vi "LSMcontroller_v58.vi"() -> ()   [LabVIEW 2015] (continued)
                    n3053 = local write "status"(w6244) -> ()
                  }
                  frame #2 {
                    n3054 = call "2pparameters.vi"("command"="get") -> ("params out"=w6274:T12)  [unwired: 1 in]
                    n3055 = Unbundle By Name(w6274) -> ("Xpixels Img"=w6273:i32, "Vx-min Img"=w6272:dbl, "VX-max Img"=w6271:dbl, "Ypixels Img"=w6270:i32, "Vy-min Img"=w6269:dbl, "Vy-max Img"=w6268:dbl, "Colormap"=w6267:u16, "square pixels"=w6266:bool, "square matrix"=w6265:bool, "Angle Img"=w6264:dbl, "Drawing Mode"=w6263:u16)
                    n3056 = local write "xpixels ref"(w6273) -> ()
                    n3057 = local write "Vx-min ref"(w6272) -> ()
                    n3058 = local write "Vx-max ref"(w6271) -> ()
                    n3059 = local write "ypixels ref"(w6270) -> ()
                    n3060 = local write "Vy-min ref"(w6269) -> ()
                    n3061 = local write "Vy-max ref"(w6268) -> ()
                    n3062 = local write "Colormap"(w6267) -> ()
                    n3063 = local write "Square pixels"(w6266) -> ()
                    n3064 = local write "square matrix"(w6265) -> ()
                    n3065 = local write "Angle ref"(w6264) -> ()
                    n3066 = local write "ROI Type"(w6263) -> ()
                    n3067 = call "2pparameters.vi"("command"="get") -> ("params out"=w6257:T12)  [unwired: 1 in]
                    n3068 = Unbundle By Name(w6257) -> ("Xpixels"=w6251:i32, "Vxminref"=w6255:dbl, "Vxmaxref"=w6254:dbl, "Ypixels"=w6250:i32, "Vyminref"=w6253:dbl, "Vymaxref"=w6252:dbl, "Colormap"=w6258:u16, "square pixels"=w6259:bool, "square matrix"=w6260:bool, "Angle draw"=w6261:dbl, "Drawing Mode"=w6262:u16)
                    n3069 = local write "Vy-max draw"(w6252) -> ()
                    n3070 = local write "Angle drawing"(w6261) -> ()
                    n3071 = local write "Colormap"(w6258) -> ()
                    n3072 = local write "Square pixels"(w6259) -> ()
                    n3073 = local write "square matrix"(w6260) -> ()
                    n3074 = local write "ROI Type"(w6262) -> ()
                    n3075 = local write "xpixels draw"(w6251) -> ()
                    n3076 = local write "ypixels draw"(w6250) -> ()
                    n3077 = local write "Vx-min draw"(w6255) -> ()
                    n3078 = local write "Vx-max draw"(w6254) -> ()
                    n3079 = local write "Vy-min draw"(w6253) -> ()
                  }
                  frame #3 {
                    n3080 = property on="ROI" class="Bool (strict)"("Val(Sgnl)"=FALSE ("x/y scan")) -> ()  [unwired: 2 in, 2 out]
                  }
                }
              }
            }
          }
          event "Xdattype": Value Change {
            n3081 = event-data() -> ()  [unwired: 1 in, 1 out]
            n3082 = case shown="True" "Xdattype" {
              frame False {
              }
              frame True {
                n3083 = stacked-sequence {
                  frame #0 {
                    n3084 = Current VI's Path() -> (path=w6287:path)
                    n3085 = Strip Path(path=w6287) -> (stripped path=w6288:path)  [unwired: 1 out]
                    n3086 = Build Path(base path=w6288, name or relative path="subVIs\\Misc\\Changedataconfig.vi") -> (appended path=w6286:path)
                    n3087 = call <vilib>:"Set Busy.vi"() -> ("error out"=w6284:errorcluster)  [unwired: 10 in, 1 out]
                    n3088 = Open VI Reference(type specifier VI Refnum (for type only)=refnum<vi> refnum, vi path=w6286, error in (no error)=w6284) -> (vi reference=w6279:refnum<vi>, error out=w6281:errorcluster)  [unwired: 3 in]
                    n3089 = call-by-ref "?"(reference=w6279, error in=w6281) -> (reference out=w6283:refnum<vi>, error out=w6282:errorcluster)  [unwired: 12 in]
                    n3090 = Close Reference(reference=w6283, error in (no error)=w6282) -> (error out=w6278:errorcluster)
                    "status" <- w6278
                    n3091 = call <vilib>:"Unset Busy.vi"("error in (no error)"=w6278) -> ()  [unwired: 10 in, 1 out]
                  }
                  frame #1 {
                    n3092 = property on="Xdattype" class="Bool (strict)"("Val(Sgnl)"=FALSE ("x/y scan")) -> ()  [unwired: 2 in, 2 out]
                  }
                }
              }
            }
          }
          event "XautoOD": Value Change {
            n3093 = event-data() -> ()  [unwired: 1 in, 1 out]
            n3094 = case shown="True" "XautoOD" {
              frame False {
              }
              frame True {
                n3095 = stacked-sequence {
                  frame #0 {
                    n3096 = Current VI's Path() -> (path=w6300:path)
                    n3097 = Strip Path(path=w6300) -> (stripped path=w6301:path)  [unwired: 1 out]
                    n3098 = Build Path(base path=w6301, name or relative path="subVIs\\Misc\\ChangeautoODs.vi") -> (appended path=w6299:path)
                    n3099 = call <vilib>:"Set Busy.vi"() -> ("error out"=w6297:errorcluster)  [unwired: 10 in, 1 out]
                    n3100 = Open VI Reference(type specifier VI Refnum (for type only)=refnum<vi> refnum, vi path=w6299, error in (no error)=w6297) -> (vi reference=w6292:refnum<vi>, error out=w6294:errorcluster)  [unwired: 3 in]
                    n3101 = call-by-ref "?"(reference=w6292, error in=w6294) -> (reference out=w6296:refnum<vi>, error out=w6295:errorcluster)  [unwired: 12 in]
                    n3102 = Close Reference(reference=w6296, error in (no error)=w6295) -> (error out=w6291:errorcluster)
                    "status 2" <- w6291
                    n3103 = call <vilib>:"Unset Busy.vi"("error in (no error)"=w6291) -> ()  [unwired: 10 in, 1 out]
                  }
                  frame #1 {
                    n3104 = property on="XautoOD" class="Bool (strict)"("Val(Sgnl)"=FALSE ("x/y scan")) -> ()  [unwired: 2 in, 2 out]
                  }
                }
              }
            }
          }
          event "SetMan": Value Change {
            n3105 = event-data() -> ()  [unwired: 1 in, 1 out]
            n3106 = case shown="True" "SetMan" {
              frame False {
              }
              frame True {
                n3107 = stacked-sequence {
                  frame #0 {
                    w6304 = u16 0 items=["Rectangle", "Circle", "Freeform Boundary", "Freeform Interior"] ("ROI Type")
                    n3108 = local write "ROI Type"(w6304) -> ()
                    n3109 = local read "Square pixels"() -> (w6310:bool)
                    n3110 = case shown="True" w6310 {
                      frame False {
                        n3111 = local read "square matrix"() -> (w6311:bool)
                        n3112 = case shown="False" w6311 {
                          frame False {
                            "ypixels ref" <- "ypixels"
                            "xpixels ref" <- "xpixels"
                          }
                          frame True {
                            n3113 = local read "xpixels"() -> (w6316:i32)
                            n3114 = local read "ypixels"() -> (w6315:i32)
                            n3115 = Max & Min(x=w6316, y=w6315) -> (max(x,y)=w6314:i32)  [unwired: 1 out]
                            n3116 = local write "xpixels ref"(w6314) -> ()
                            n3117 = local write "ypixels ref"(w6314) -> ()
                          }
                        }
                      }
                      frame True {
                        n3118 = local read "square matrix"() -> (w6317:bool)
                        n3119 = case shown="False" w6317 {
                          frame False {
                            n3120 = local read "Vxmax"() -> (w6331:dbl)
                            n3121 = local read "Vx-min"() -> (w6330:dbl)
                            n3122 = local read "Vy-max"() -> (w6326:dbl)
                            n3123 = local read "Vy-min"() -> (w6327:dbl)
                            n3124 = Subtract(x=w6326, y=w6327) -> (x-y=w6328:dbl)
                            n3125 = Subtract(x=w6331, y=w6330) -> (x-y=w6329:dbl)
                            n3126 = Absolute Value(x=w6328) -> (abs(x)=w6319:dbl)
                            n3127 = Absolute Value(x=w6329) -> (abs(x)=w6320:dbl)
                            n3128 = Divide(x=w6320, y=w6319) -> (x/y=w6325:dbl)
                            n3129 = Greater Or Equal?(x=w6320, y=w6319) -> (x >= y?=w6318:bool)
                            n3130 = local read "xpixels"() -> (w6324:i32)
                            n3131 = local read "ypixels"() -> (w6321:i32)
                            n3132 = case shown="False" w6318 {
                              tunnel: w6325 -> [w6336 w6339]
                              tunnel: w6324 -> [w6333 _]
                              tunnel: [w6333 w6338] -> w6323
                              tunnel: [w6332 w6337] -> w6322
                              tunnel: w6321 -> [_ w6337]
                              frame False {
                                n3133 = To Double Precision Float(number=w6333) -> (double precision float=w6335:dbl)
                                n3134 = Divide(x=w6335, y=w6336) -> (x/y=w6334:dbl)
                                n3135 = To Long Integer(number=w6334) -> (32bit integer=w6332:i32)
                              }
                              frame True {
                                n3136 = To Double Precision Float(number=w6337) -> (double precision float=w6341:dbl)
                                n3137 = Multiply(x=w6341, y=w6339) -> (x*y=w6340:dbl)
                                n3138 = To Long Integer(number=w6340) -> (32bit integer=w6338:i32)
                              }
                            }
                            n3139 = local write "ypixels ref"(w6322) -> ()
                            n3140 = local write "xpixels ref"(w6323) -> ()
                          }
                          frame True {
                          }
                        }
                      }
                    }
                    "Vx-max ref" <- "Vxmax"
                    "Vx-min ref" <- "Vx-min"
                    "Vy-max ref" <- "Vy-max"
                    "Vy-min ref" <- "Vy-min"
                    "Angle ref" <- "Angle"
                  }
                  frame #1 {
                    n3141 = property on="SetMan" class="Bool (strict)"("Val(Sgnl)"=FALSE ("Value (Signaling)")) -> ()  [unwired: 2 in, 2 out]
                  }
                }
              }
            }
          }
          event "SetMan 2": Value Change {
            n3142 = event-data() -> ()  [unwired: 1 in, 1 out]
            n3143 = case shown="True" "SetMan 2" {
              frame False {
              }
              frame True {
                n3144 = stacked-sequence {
                  frame #0 {
                    n3145 = local write "Vx-ref"("Vx") -> ()
                    n3146 = local write "Vy-ref"("Vy") -> ()
                  }
                  frame #1 {
                    n3147 = property on="SetMan 2" class="Bool (strict)"("Val(Sgnl)"=FALSE ("Value (Signaling)")) -> ()  [unwired: 2 in, 2 out]
                  }
                }
              }
            }
          }
          event "Reset Coords": Value Change {
            n3148 = event-data() -> ("NewVal"=w6347:bool)  [unwired: 1 in, 5 out]
            n3149 = case shown="True" w6347 {
              frame False {
              }
              frame True {
                n3150 = stacked-sequence {
                  frame #0 {
                    n3151 = local write "xpixels"(256 ("xpixels")) -> ()
                    n3152 = local write "ypixels"(256 ("ypixels")) -> ()
                    n3153 = local write "Vxmax"(9.0 ("Vx-max")) -> ()
                    n3154 = local write "Vx-min"(-9.0 ("Vx-min")) -> ()
                    n3155 = local write "Vy-max"(9.0 ("Vy-max")) -> ()
                    n3156 = local write "Vy-min"(-9.0 ("Vy-min")) -> ()
                    n3157 = local write "Angle"(0.0 ("Angle")) -> ()
                  }
                  frame #1 {
                    n3158 = property on="Reset Coords" class="Bool (strict)"("Value"=FALSE ("TROI")) -> ()  [unwired: 2 in, 2 out]
                  }
                }
              }
            }
          }
          event "TROI": Value Change {
            n3159 = event-data() -> ()  [unwired: 1 in, 1 out]
            n3160 = case shown="True" "TROI" {
              frame False {
              }
              frame True {
                n3161 = stacked-sequence {
                  frame #0 {
                    n3162 = local read "Vy-min ref"() -> (w6361:dbl)
                    n3163 = local read "Vy-max ref"() -> (w6360:dbl)
                    n3164 = local read "Vx-max ref"() -> (w6358:dbl)
                    n3165 = local read "Vx-min ref"() -> (w6359:dbl)
                    n3166 = local read "ypixels ref"() -> (w6363:i32)
                    n3167 = local read "xpixels ref"() -> (w6362:i32)
                    n3168 = local read "Angle ref"() -> (w6357:dbl)
                    n3169 = local write "Angle"(w6357) -> ()
                    n3170 = local write "xpixels"(w6362) -> ()
                    n3171 = local write "Vy-min"(w6361) -> ()
                    n3172 = local write "Vy-max"(w6360) -> ()
                    n3173 = local write "Vx-min"(w6359) -> ()
                    n3174 = local write "ypixels"(w6363) -> ()
                    n3175 = local write "Vxmax"(w6358) -> ()
                  }
                  frame #1 {
                    n3176 = property on="TROI" class="Bool (strict)"("Value"=FALSE ("TROI")) -> ()  [unwired: 2 in, 2 out]
                  }
                }
              }
            }
          }
          event "TROI 2": Value Change {
            n3177 = event-data() -> ()  [unwired: 1 in, 1 out]
            n3178 = case shown="True" "TROI 2" {
              frame False {
              }
              frame True {
                n3179 = stacked-sequence {
                  frame #0 {
                    n3180 = local read "Vx-ref"() -> (w6366:dbl)
                    n3181 = local read "Vy-ref"() -> (w6367:dbl)
                    n3182 = local write "Vx"(w6366) -> ()
                    n3183 = local write "Vy"(w6367) -> ()
                  }
                  frame #1 {
                    n3184 = property on="TROI 2" class="Bool (strict)"("Value"=FALSE ("TROI")) -> ()  [unwired: 2 in, 2 out]
                  }
                }
              }
            }
          }
          event "Square pixels": Value Change {
            n3185 = event-data() -> ()  [unwired: 1 in, 1 out]
            n3186 = case shown="True" "Square pixels" {
              frame False {
              }
              frame True {
                n3187 = property on="square matrix" class="Bool (strict)"("Value"=FALSE ("square matrix")) -> ()  [unwired: 2 in, 2 out]
                n3188 = property on="Square pixels" class="Bool (strict)"("Value"=TRUE ("square matrix")) -> ()  [unwired: 2 in, 2 out]
              }
            }
          }
          event "square matrix": Value Change {
            n3189 = event-data() -> ()  [unwired: 1 in, 1 out]
            n3190 = case shown="True" "square matrix" {
              frame False {
              }
              frame True {
                n3191 = property on="square matrix" class="Bool (strict)"("Value"=TRUE ("square matrix")) -> ()  [unwired: 2 in, 2 out]
                n3192 = property on="Square pixels" class="Bool (strict)"("Value"=FALSE ("square matrix")) -> ()  [unwired: 2 in, 2 out]
              }
            }
          }
          event "up", "downright", "down", "downleft", "right", "left", "upright", "upleft": Value Change {
            n3193 = event-data() -> ()  [unwired: 1 in, 6 out]
            n3194 = local read "downright"() -> (w6380:bool)
            n3195 = local read "downleft"() -> (w6382:bool)
            n3196 = local read "upright"() -> (w6378:bool)
            n3197 = local read "upleft"() -> (w6376:bool)
            n3198 = local read "down"() -> (w6381:bool)
            n3199 = local read "right"() -> (w6379:bool)
            n3200 = local read "left"() -> (w6383:bool)
            n3201 = local read "up"() -> (w6377:bool)
            n3202 = Compound Arithmetic op=OR(w6376, w6377, w6378, w6379, w6380, w6381, w6382, w6383) -> (w6375:bool)
            n3203 = case shown="True" w6375 {
              frame False {
              }
              frame True {
                n3204 = stacked-sequence {
                  frame #0 {
                    n3205 = local read "downright"() -> (w6385:bool)
                    n3206 = local read "downleft"() -> (w6387:bool)
                    n3207 = local read "BigSmall"() -> (w6384:bool)
                    n3208 = local read "upright"() -> (w6389:bool)
                    n3209 = local read "upleft"() -> (w6392:bool)
                    n3210 = local read "down"() -> (w6388:bool)
                    n3211 = local read "right"() -> (w6390:bool)
                    n3212 = local read "left"() -> (w6386:bool)
                    n3213 = local read "up"() -> (w6391:bool)
                    n3214 = call "movestageparams.vi"("command"="get") -> ("Params out"=w6395:T22)  [unwired: 1 in]
                    n3215 = Bundle By Name(cluster=w6395, "upleft"=w6392, "up"=w6391, "upright"=w6389, "right"=w6390, "downright"=w6385, "down"=w6388, "downleft"=w6387, "left"=w6386, "Bigsmall"=w6384) -> (w6396:T22)
                    n3216 = call "movestageparams.vi"("Params in"=w6396, "command"="set") -> ()  [unwired: 1 out]
                  }
                  frame #1 {
                    n3217 = disable-structure shown="Disabled" {
                      frame Disabled {
                        n3218 = call "configuration.vi"("command"="get") -> ("config out"=w6399:T13)  [unwired: 2 in, 1 out]
                        n3219 = in-place {
                          n3220 = in-place-cluster #45(w6399) -> ()  [unwired: 2 out]
                          n3221 = in-place-cluster #45("StageL"="StageL", "StageS"="StageS") -> (w6397:T13)
                        }
                        n3222 = call "configuration.vi"("config in"=w6397, "command"="set") -> ()  [unwired: 1 in, 2 out]
                      }
                      frame Enabled {
                      }
                    }
                  }
                  frame #2 {
                    n3223 = call "movestage.vi"() -> ()  [unwired: 12 in]
                  }
                  frame #3 {
                    w6403 = FALSE ("OK Button")
                    w6404 = FALSE ("OK Button")
                    n3224 = property on="down" class="Bool (strict)"("Value"=w6404) -> ()  [unwired: 2 in, 2 out]
                    n3225 = property on="up" class="Bool (strict)"("Value"=w6404) -> ()  [unwired: 2 in, 2 out]
                    n3226 = property on="right" class="Bool (strict)"("Value"=w6404) -> ()  [unwired: 2 in, 2 out]
                    n3227 = property on="left" class="Bool (strict)"("Value"=w6404) -> ()  [unwired: 2 in, 2 out]
                    n3228 = property on="upright" class="Bool (strict)"("Value"=w6403) -> ()  [unwired: 2 in, 2 out]
                    n3229 = property on="downleft" class="Bool (strict)"("Value"=w6403) -> ()  [unwired: 2 in, 2 out]
                    n3230 = property on="downright" class="Bool (strict)"("Value"=w6403) -> ()  [unwired: 2 in, 2 out]
                    n3231 = property on="upleft" class="Bool (strict)"("Value"=w6403) -> ()  [unwired: 2 in, 2 out]
                  }
                }
              }
            }
          }
          event "finite samples": Value Change {
            n3232 = event-data() -> ("NewVal"=w6405:bool)  [unwired: 1 in]
            n3233 = flat-sequence {
              tunnel: w6405 -> [w6406]
              frame #0 {
                n3234 = case shown="True" w6406 {
                  frame False {
                    w6407 = FALSE ("wavdet")
                    n3235 = property on="continuous" class="Bool (strict)"("Value"=TRUE ("continuous for display")) -> ()  [unwired: 2 in, 2 out]
                    n3236 = property on="wavdet" class="Bool (strict)"("Value"=w6407) -> ()  [unwired: 2 in, 2 out]
                    n3237 = property on="save\ndata" class="Bool (strict)"("Value"=w6407) -> ()  [unwired: 2 in, 2 out]
                    n3238 = property on="# of frames" class="DigNum (strict)"("DisabledEnum"=T8."Disabled and Grayed Out" ("Disabled")) -> ()  [unwired: 2 in, 2 out]
                    n3239 = property on="save\ndata" class="Bool (strict)"("DisabledEnum"=T8."Disabled and Grayed Out" ("Disabled")) -> ()  [unwired: 2 in, 2 out]
                    "Save tab" <- enum32{"withsave", "withoutsave"}."withsave" ("Save tab")
                  }
                  frame True {
                    w6414 = FALSE ("continuous for display")
                    n3240 = property on="continuous" class="Bool (strict)"("Value"=w6414) -> ()  [unwired: 2 in, 2 out]
                    n3241 = property on="wavdet" class="Bool (strict)"("Value"=w6414) -> ()  [unwired: 2 in, 2 out]
                    n3242 = local write "Save tab"(enum32{"withsave", "withoutsave"}."withsave" ("Save tab")) -> ()
                    n3243 = property on="save\ndata" class="Bool (strict)"("DisabledEnum"=T8."Enabled" ("Disabled")) -> ()  [unwired: 2 in, 2 out]
                    n3244 = property on="save\ndata" class="Bool (strict)"("Value"=TRUE ("save\ndata")) -> ()  [unwired: 2 in, 2 out]
                    n3245 = property on="# of frames" class="DigNum (strict)"("DisabledEnum"=T8."Enabled" ("Disabled")) -> ()  [unwired: 2 in, 2 out]
                  }
                }
              }
              frame #1 {
                n3246 = local read "finite samples"() -> (w6423:bool)
                n3247 = local read "continuous"() -> (w6422:bool)
                n3248 = local read "wavdet"() -> (w6421:bool)
                n3249 = call "2pparameters.vi"("command"="get") -> ("params out"=w6417:T12)  [unwired: 1 in]
                n3250 = Bundle By Name(cluster=w6417, "finite"=w6423, "cont"=w6422, "wavdet"=w6421) -> (w6420:T12)
                n3251 = call "2pparameters.vi"("Params in"=w6420, "command"="set") -> ()  [unwired: 1 out]
              }
            }
          }
          event "continuous": Value Change {
            n3252 = event-data() -> ("NewVal"=w6424:bool)  [unwired: 1 in]
            n3253 = flat-sequence {
              tunnel: w6424 -> [w6425]
              frame #0 {
                n3254 = case shown="True" w6425 {
                  frame False {
                    n3255 = property on="finite samples" class="Bool (strict)"("Value"=TRUE ("finite samples for recording")) -> ()  [unwired: 2 in, 2 out]
                    n3256 = property on="save\ndata" class="Bool (strict)"("Value"=TRUE ("save\ndata")) -> ()  [unwired: 2 in, 2 out]
                    n3257 = property on="wavdet" class="Bool (strict)"("Value"=FALSE ("wavdet")) -> ()  [unwired: 2 in, 2 out]
                    n3258 = local write "Save tab"(enum32{"withsave", "withoutsave"}."withsave" ("Save tab")) -> ()
                    n3259 = property on="# of frames" class="DigNum (strict)"("DisabledEnum"=T8."Enabled" ("Disabled")) -> ()  [unwired: 2 in, 2 out]
                    n3260 = property on="save\ndata" class="Bool (strict)"("DisabledEnum"=T8."Enabled" ("Disabled")) -> ()  [unwired: 2 in, 2 out]
                  }
                  frame True {
                    w6432 = FALSE ("finite samples for recording")
                    n3261 = property on="finite samples" class="Bool (strict)"("Value"=w6432) -> ()  [unwired: 2 in, 2 out]
                    n3262 = property on="wavdet" class="Bool (strict)"("Value"=w6432) -> ()  [unwired: 2 in, 2 out]
                    n3263 = property on="save\ndata" class="Bool (strict)"("Value"=w6432) -> ()  [unwired: 2 in, 2 out]
                    n3264 = local write "Save tab"(enum32{"withsave", "withoutsave"}."withsave" ("Save tab")) -> ()
                    n3265 = property on="# of frames" class="DigNum (strict)"("DisabledEnum"=T8."Disabled and Grayed Out" ("Disabled")) -> ()  [unwired: 2 in, 2 out]
                    n3266 = property on="save\ndata" class="Bool (strict)"("DisabledEnum"=T8."Disabled and Grayed Out" ("Disabled")) -> ()  [unwired: 2 in, 2 out]
                  }
                }
              }
              frame #1 {
                n3267 = local read "finite samples"() -> (w6442:bool)
                n3268 = local read "continuous"() -> (w6441:bool)
                n3269 = local read "wavdet"() -> (w6440:bool)
                n3270 = call "2pparameters.vi"("command"="get") -> ("params out"=w6436:T12)  [unwired: 1 in]
                n3271 = Bundle By Name(cluster=w6436, "finite"=w6442, "cont"=w6441, "wavdet"=w6440) -> (w6439:T12)
                n3272 = call "2pparameters.vi"("Params in"=w6439, "command"="set") -> ()  [unwired: 1 out]
              }
            }
          }
          event "wavdet": Value Change {
            n3273 = event-data() -> ("NewVal"=w6443:bool)  [unwired: 1 in]
            n3274 = flat-sequence {
              tunnel: w6443 -> [w6444]
              frame #0 {
                n3275 = case shown="False" w6444 {
                  frame False {
                    n3276 = property on="finite samples" class="Bool (strict)"("Value"=TRUE ("finite samples for recording")) -> ()  [unwired: 2 in, 2 out]
                    n3277 = property on="continuous" class="Bool (strict)"("Value"=FALSE ("continuous")) -> ()  [unwired: 2 in, 2 out]
                    n3278 = local write "Save tab"(enum32{"withsave", "withoutsave"}."withsave" ("Save tab")) -> ()
                    n3279 = property on="save\ndata" class="Bool (strict)"("DisabledEnum"=T8."Enabled" ("Disabled")) -> ()  [unwired: 2 in, 2 out]
                    n3280 = property on="# of frames" class="DigNum (strict)"("DisabledEnum"=T8."Enabled" ("Disabled")) -> ()  [unwired: 2 in, 2 out]
                    n3281 = property on="save\ndata" class="Bool (strict)"("Value"=TRUE ("save\ndata")) -> ()  [unwired: 2 in, 2 out]
                  }
                  frame True {
                    w6453 = FALSE ("finite samples for recording")
                    n3282 = property on="finite samples" class="Bool (strict)"("Value"=w6453) -> ()  [unwired: 2 in, 2 out]
                    n3283 = property on="continuous" class="Bool (strict)"("Value"=w6453) -> ()  [unwired: 2 in, 2 out]
                    n3284 = property on="save\ndata" class="Bool (strict)"("DisabledEnum"=T8."Enabled" ("Disabled")) -> ()  [unwired: 2 in, 2 out]
                    n3285 = local write "Save tab"(enum32{"withsave", "withoutsave"}."withsave" ("Save tab")) -> ()
                    n3286 = property on="# of frames" class="DigNum (strict)"("DisabledEnum"=T8."Disabled" ("Disabled")) -> ()  [unwired: 2 in, 2 out]
                    n3287 = property on="save\ndata" class="Bool (strict)"("Value"=TRUE ("save\ndata")) -> ()  [unwired: 2 in, 2 out]
                  }
                }
              }
              frame #1 {
                n3288 = local read "finite samples"() -> (w6456:bool)
                n3289 = local read "continuous"() -> (w6457:bool)
                n3290 = local read "wavdet"() -> (w6458:bool)
                n3291 = call "2pparameters.vi"("command"="get") -> ("params out"=w6462:T12)  [unwired: 1 in]
                n3292 = Bundle By Name(cluster=w6462, "finite"=w6456, "cont"=w6457, "wavdet"=w6458) -> (w6459:T12)
                n3293 = call "2pparameters.vi"("Params in"=w6459, "command"="set") -> ()  [unwired: 1 out]
              }
            }
          }
          event "cursors": Value Change {
            n3294 = event-data() -> ()  [unwired: 1 in, 5 out]
            n3295 = case shown="True" "cursors" {
              frame False {
                n3296 = property on="img_CH1" class="IntGraph (strict)"("Active Cursor"=u32 0, "Cursor.Cursor Style"=u8 0 ("Cursor Style"), "Cursor.Cursor Point Style"=u8 0 ("Cursor Point Style")) -> ("Cursor.Cursor Position:Cursor X"=w6467:dbl, "Cursor.Cursor Position:Cursor Y"=w6468:dbl)  [unwired: 2 in, 2 out]
                n3297 = property on="img_CH2" class="IntGraph (strict)"("Active Cursor"=u32 0, "Cursor.Cursor Style"=u8 0 ("Cursor Style"), "Cursor.Cursor Point Style"=u8 0 ("Cursor Point Style")) -> ()  [unwired: 2 in, 2 out]
                n3298 = local write "cursor x [pixel]"(w6467) -> ()
                n3299 = local write "cursor y [pixel]"(w6468) -> ()
              }
              frame True {
                n3300 = stacked-sequence {
                  frame #0 {
                    n3301 = call "2pparameters.vi"("command"="get") -> ("params out"=w6483:T12)  [unwired: 1 in]
                    n3302 = Unbundle By Name(w6483) -> ("Xpixels Img"=w6484:i32, "Ypixels Img"=w6481:i32)
                    n3303 = To Double Precision Float(number=w6481) -> (double precision float=w6475:dbl)
                    n3304 = To Double Precision Float(number=w6484) -> (double precision float=w6480:dbl)
                    n3305 = Divide(x=w6475, y=2.0) -> (x/y=w6476:dbl)
                    n3306 = Divide(x=w6480, y=2.0) -> (x/y=w6478:dbl)
                    n3307 = Round To Nearest(number=w6476) -> (nearest integer value=w6474:dbl)
                    n3308 = Round To Nearest(number=w6478) -> (nearest integer value=w6477:dbl)
                    n3309 = property on="img_CH1" class="IntGraph (strict)"("Active Cursor"=u32 0, "Cursor.Cursor Style"=u8 8 ("Cursor Style"), "Cursor.Cursor Point Style"=u8 5 ("Cursor Point Style"), "Cursor.Cursor Position:Cursor X"=w6477, "Cursor.Cursor Position:Cursor Y"=w6474, "Cursor.Visible"=TRUE) -> ()  [unwired: 2 in, 2 out]
                  }
                  frame #1 {
                    n3310 = call "2pparameters.vi"("command"="get") -> ("params out"=w6503:T12)  [unwired: 1 in]
                    n3311 = call "2pparameters.vi"("command"="get") -> ("params out"=w6501:T12)  [unwired: 1 in]
                    n3312 = property on="img_CH1" class="IntGraph (strict)"("Active Cursor"=u32 0, "Cursor.Cursor Style"=u8 8 ("Cursor Style"), "Cursor.Cursor Point Style"=u8 5 ("Cursor Point Style")) -> ("Cursor.Cursor Position:Cursor X"=w6496:dbl, "Cursor.Cursor Position:Cursor Y"=w6495:dbl, "Cursor.Cursor Index"=w6518:i32, "Cursor.Cursor Plot"=w6517:i32, "Cursor.Visible"=w6488:bool)  [unwired: 2 in, 2 out]
                    "cursor x [pixel]" <- w6496
                    "cursor y [pixel]" <- w6495
                    n3313 = Unbundle By Name(w6503) -> ("Vy-max Img"=w6505:dbl, "Vy-min Img"=w6492:dbl, "Ypixels Img"=w6507:i32)
                    n3314 = Unbundle By Name(w6501) -> ("VX-max Img"=w6502:dbl, "Vx-min Img"=w6490:dbl, "Xpixels Img"=w6506:i32)
                    n3315 = Subtract(x=w6505, y=w6492) -> (x-y=w6510:dbl)
                    n3316 = Subtract(x=w6502, y=w6490) -> (x-y=w6508:dbl)
                    n3317 = local read "img_CH2"() -> (w6514:sgl[][])
                    n3318 = To Double Precision Float(number=w6506) -> (double precision float=w6509:dbl)
                    n3319 = local read "img_CH1"() -> (w6515:sgl[][])
                    n3320 = To Double Precision Float(number=w6507) -> (double precision float=w6511:dbl)
                    n3321 = Index Array(array=w6515, index (row)=w6518, index (col)=w6517) -> (element=→"value CH 1":sgl)
                    n3322 = Index Array(array=w6514, index (row)=w6518, index (col)=w6517) -> (element=→"value CH 2":sgl)
                    n3323 = Divide(x=w6508, y=w6509) -> (x/y=w6512:dbl)
                    n3324 = Divide(x=w6510, y=w6511) -> (x/y=w6513:dbl)
                    n3325 = Multiply(x=w6496, y=w6512) -> (x*y=w6491:dbl)
                    n3326 = Multiply(x=w6495, y=w6513) -> (x*y=w6494:dbl)
                    n3327 = property on="img_CH2" class="IntGraph (strict)"("Active Cursor"=u32 0, "Cursor.Cursor Style"=u8 8 ("Cursor Style"), "Cursor.Cursor Point Style"=u8 5 ("Cursor Point Style"), "Cursor.Cursor Position:Cursor X"=w6496, "Cursor.Cursor Position:Cursor Y"=w6495, "Cursor.Visible"=w6488) -> ()  [unwired: 2 in, 2 out]
                    n3328 = Add(x=w6491, y=w6490) -> (x+y=w6489:dbl)
                    n3329 = Add(x=w6494, y=w6492) -> (x+y=w6493:dbl)
                    n3330 = local write "Vx-ref"(w6489) -> ()
                    n3331 = local write "Vy-ref"(w6493) -> ()
                  }
                }
              }
            }
          }
          event "img_CH1": Cursor Move {
            n3332 = event-data() -> ("CursIdx"=w6523:i32)  [unwired: 1 in]
            n3333 = Equal To 0?(x=w6523) -> (x = 0?=w6524:bool)
            n3334 = case shown="True" w6524 {
              frame False {
              }
              frame True {
                n3335 = call "2pparameters.vi"("command"="get") -> ("params out"=w6544:T12)  [unwired: 1 in]
                n3336 = call "2pparameters.vi"("command"="get") -> ("params out"=w6546:T12)  [unwired: 1 in]
                n3337 = property on="img_CH1" class="IntGraph (strict)"("Active Cursor"=u32 0, "Cursor.Cursor Style"=u8 8 ("Cursor Style"), "Cursor.Cursor Point Style"=u8 5 ("Cursor Point Style")) -> ("Cursor.Cursor Position:Cursor X"=w6533:dbl, "Cursor.Cursor Position:Cursor Y"=w6532:dbl, "Cursor.Cursor Plot"=w6552:i32, "Cursor.Cursor Index"=w6551:i32, "Cursor.Visible"=w6525:bool)  [unwired: 2 in, 2 out]
                n3338 = Unbundle By Name(w6544) -> ("Vy-max Img"=w6542:dbl, "Vy-min Img"=w6531:dbl, "Ypixels Img"=w6540:i32)
                n3339 = Unbundle By Name(w6546) -> ("VX-max Img"=w6545:dbl, "Vx-min Img"=w6526:dbl, "Xpixels Img"=w6541:i32)
                n3340 = Subtract(x=w6542, y=w6531) -> (x-y=w6537:dbl)
                n3341 = Subtract(x=w6545, y=w6526) -> (x-y=w6539:dbl)
                n3342 = local write "cursor x [pixel]"(w6533) -> ()
                n3343 = local write "cursor y [pixel]"(w6532) -> ()
                n3344 = To Double Precision Float(number=w6541) -> (double precision float=w6538:dbl)
                n3345 = To Double Precision Float(number=w6540) -> (double precision float=w6536:dbl)
                n3346 = local read "img_CH2"() -> (w6553:sgl[][])
                n3347 = local read "img_CH1"() -> (w6556:sgl[][])
                n3348 = Index Array(array=w6553, index (row)=w6552, index (col)=w6551) -> (element=w6554:sgl)
                n3349 = Index Array(array=w6556, index (row)=w6552, index (col)=w6551) -> (element=w6555:sgl)
                n3350 = Divide(x=w6539, y=w6538) -> (x/y=w6535:dbl)
                n3351 = Divide(x=w6537, y=w6536) -> (x/y=w6534:dbl)
                n3352 = local write "value CH 2"(w6554) -> ()
                n3353 = Multiply(x=w6533, y=w6535) -> (x*y=w6528:dbl)
                n3354 = local write "value CH 1"(w6555) -> ()
                n3355 = Multiply(x=w6532, y=w6534) -> (x*y=w6530:dbl)
                n3356 = Add(x=w6528, y=w6526) -> (x+y=w6527:dbl)
                n3357 = local write "Vx-ref"(w6527) -> ()
                n3358 = Add(x=w6530, y=w6531) -> (x+y=w6529:dbl)
                n3359 = property on="img_CH2" class="IntGraph (strict)"("Active Cursor"=u32 0, "Cursor.Cursor Style"=u8 8 ("Cursor Style"), "Cursor.Cursor Point Style"=u8 5 ("Cursor Point Style"), "Cursor.Cursor Position:Cursor X"=w6533, "Cursor.Cursor Position:Cursor Y"=w6532, "Cursor.Visible"=w6525) -> ()  [unwired: 2 in, 2 out]
                n3360 = local write "Vy-ref"(w6529) -> ()
              }
            }
          }
          event "img_CH2": Cursor Move {
            n3361 = event-data() -> ("CursIdx"=w6560:i32)  [unwired: 1 in]
            n3362 = Equal To 0?(x=w6560) -> (x = 0?=w6561:bool)
            n3363 = case shown="True" w6561 {
              frame False {
              }
              frame True {
                n3364 = property on="img_CH2" class="IntGraph (strict)"("Active Cursor"=u32 0, "Cursor.Cursor Style"=u8 8 ("Cursor Style"), "Cursor.Cursor Point Style"=u8 5 ("Cursor Point Style")) -> ("Cursor.Cursor Position:Cursor X"=w6569:dbl, "Cursor.Cursor Position:Cursor Y"=w6570:dbl, "Cursor.Cursor Plot"=w6589:i32, "Cursor.Cursor Index"=w6588:i32, "Cursor.Visible"=w6562:bool)  [unwired: 2 in, 2 out]
                n3365 = call "2pparameters.vi"("command"="get") -> ("params out"=w6581:T12)  [unwired: 1 in]
                n3366 = call "2pparameters.vi"("command"="get") -> ("params out"=w6583:T12)  [unwired: 1 in]
                n3367 = local read "img_CH1"() -> (w6593:sgl[][])
                n3368 = local read "img_CH2"() -> (w6590:sgl[][])
                n3369 = local write "cursor x [pixel]"(w6569) -> ()
                n3370 = local write "cursor y [pixel]"(w6570) -> ()
                n3371 = Unbundle By Name(w6581) -> ("Vy-max Img"=w6579:dbl, "Vy-min Img"=w6564:dbl, "Ypixels Img"=w6577:i32)
                n3372 = Unbundle By Name(w6583) -> ("VX-max Img"=w6582:dbl, "Vx-min Img"=w6567:dbl, "Xpixels Img"=w6578:i32)
                n3373 = Index Array(array=w6593, index (row)=w6589, index (col)=w6588) -> (element=w6592:sgl)
                n3374 = Index Array(array=w6590, index (row)=w6589, index (col)=w6588) -> (element=w6591:sgl)
                n3375 = local write "value CH 2"(w6591) -> ()
                n3376 = local write "value CH 1"(w6592) -> ()
                n3377 = Subtract(x=w6579, y=w6564) -> (x-y=w6574:dbl)
                n3378 = Subtract(x=w6582, y=w6567) -> (x-y=w6576:dbl)
                n3379 = To Double Precision Float(number=w6578) -> (double precision float=w6575:dbl)
                n3380 = To Double Precision Float(number=w6577) -> (double precision float=w6573:dbl)
                n3381 = Divide(x=w6576, y=w6575) -> (x/y=w6572:dbl)
                n3382 = Divide(x=w6574, y=w6573) -> (x/y=w6571:dbl)
                n3383 = Multiply(x=w6569, y=w6572) -> (x*y=w6568:dbl)
                n3384 = Multiply(x=w6570, y=w6571) -> (x*y=w6565:dbl)
                n3385 = property on="img_CH1" class="IntGraph (strict)"("Active Cursor"=u32 0, "Cursor.Cursor Style"=u8 8 ("Cursor Style"), "Cursor.Cursor Point Style"=u8 5 ("Cursor Point Style"), "Cursor.Cursor Position:Cursor X"=w6569, "Cursor.Cursor Position:Cursor Y"=w6570, "Cursor.Visible"=w6562) -> ()  [unwired: 2 in, 2 out]
                n3386 = Add(x=w6568, y=w6567) -> (x+y=→"Vx-ref":dbl)
                n3387 = Add(x=w6565, y=w6564) -> (x+y=→"Vy-ref":dbl)
              }
            }
          }
          event "auto shutter": Value Change {
            n3388 = event-data() -> ()  [unwired: 1 in, 6 out]
            n3389 = call "2pparameters.vi"("command"="get") -> ("params out"=w6599:T12)  [unwired: 1 in]
            n3390 = in-place {
              n3391 = in-place-cluster #46(w6599) -> ()  [unwired: 1 out]
              n3392 = local read "auto shutter"() -> (w6601:bool)
              n3393 = in-place-cluster #46("autoshutter"=w6601) -> (w6597:T12)
            }
            n3394 = call "2pparameters.vi"("Params in"=w6597, "command"="set") -> ()  [unwired: 1 out]
          }
          event "auto OD": Value Change {
            n3395 = event-data() -> ()  [unwired: 1 in, 6 out]
            n3396 = call "2pparameters.vi"("command"="get") -> ("params out"=w6604:T12)  [unwired: 1 in]
            n3397 = in-place {
              n3398 = in-place-cluster #47(w6604) -> ()  [unwired: 1 out]
              n3399 = local read "auto OD"() -> (w6606:bool)
              n3400 = in-place-cluster #47("auto OD"=w6606) -> (w6602:T12)
            }
            n3401 = call "2pparameters.vi"("Params in"=w6602, "command"="set") -> ()  [unwired: 1 out]
          }
          event "ODfilt": Value Change {
            n3402 = event-data() -> ("OldVal"=w6607:u16)  [unwired: 1 in, 5 out]
            n3403 = local read "ODfilt"() -> (w6608:u16)
            n3404 = call "2pparameters.vi"("command"="get") -> ("params out"=w6611:T12)  [unwired: 1 in]
            n3405 = call "filterwheelcontrol_nothorlabslib.vi"("Current OD filt"=w6607, "New ODfilt"=w6608) -> ()  [unwired: 1 in]
            n3406 = in-place {
              in-place-border: w6608 -> [w6613]
              n3407 = in-place-cluster #48(w6611) -> ()  [unwired: 1 out]
              n3408 = in-place-cluster #48("ODfilt"=w6613) -> (w6609:T12)
            }
            n3409 = call "2pparameters.vi"("Params in"=w6609, "command"="set") -> ()  [unwired: 1 out]
          }
          event "Exit": Value Change {
            n3410 = event-data() -> ()  [unwired: 1 in, 5 out]
          }
        }
        n3411 = Wait (ms)(milliseconds to wait=u32 50) -> ()  [unwired: 1 out]
      }
      n3412 = while {
        stop <- w75 stop-if-true
        # "Waveform generation"
        n3413 = event shown="[1] \"Add AO wave\": Value Change" {
          selector: _ -> [_ _ _ _ _ _ _ _ _ _ _ _ _ _ _ _ _]
          dyn-events: _ -> [_ _ _ _ _ _ _ _ _ _ _ _ _ _ _ _ _]
          timeout: _ -> [_ _ _ _ _ _ _ _ _ _ _ _ _ _ _ _ _]
          tunnel: [_ _ _ _ _ _ _ _ _ _ _ _ _ _ _ _ w2048] -> w75
          event Timeout {
            n3414 = event-data() -> ()  [unwired: 1 in, 3 out]
          }
          event "Add AO wave": Value Change {
            n3415 = event-data() -> ("NewVal"=w76:bool)  [unwired: 1 in, 5 out]
            n3416 = case shown="True" w76 {
              frame False {
              }
              frame True {
                n3417 = stacked-sequence {
                  frame #0 {
                    n3418 = local read "Measurement"() -> (w77:T5)
                    n3419 = case shown="\"Lifetime (contour)\"" w77 {
                      frame "X-Y-t movie", Default {
                        n3420 = local read "avpp"() -> (w98:i32)
                        n3421 = local read "Angle ref"() -> (w97:dbl)
                        n3422 = local read "ROI Type"() -> (w96:u16)
                        n3423 = local read "xpixels ref"() -> (w93:i32)
                        n3424 = local read "Vx-min ref"() -> (w92:dbl)
                        n3425 = local read "Vx-max ref"() -> (w91:dbl)
                        n3426 = local read "ypixels ref"() -> (w89:i32)
                        n3427 = local read "Vy-min ref"() -> (w90:dbl)
                        n3428 = local read "Vy-max ref"() -> (w86:dbl)
                        n3429 = local read "Sampling rate"() -> (w80:dbl)
                        n3430 = local read "finite samples"() -> (w81:bool)
                        n3431 = local read "continuous"() -> (w84:bool)
                        n3432 = local read "wavdet"() -> (w85:bool)
                        n3433 = local read "# of frames"() -> (w83:i32)
                        n3434 = local read "maxbufferAI"() -> (w82:i32)
                        n3435 = local read "Override AI buffer"() -> (w78:bool)
                        n3436 = call "2pparameters.vi"("command"="get") -> ("params out"=w95:T12)  [unwired: 1 in]
                        n3437 = Bundle By Name(cluster=w95, "type"="X-Y-t movie", "avpp"=w98, "Angle Img"=w97, "Xpixels Img"=w93, "Vx-min Img"=w92, "VX-max Img"=w91, "Ypixels Img"=w89, "Vy-min Img"=w90, "Vy-max Img"=w86, "srate"=w80, "srate Img"=w80, "finite"=w81, "cont"=w84, "wavdet"=w85, "measpoints"=w83, "maxbufferAI"=w82, "Drawing Mode"=w96, "Vz-reset"=0.0, "AIoverride"=w78) -> (w87:T12)
                        n3438 = call "2pparameters.vi"("Params in"=w87, "command"="set") -> ()  [unwired: 1 out]
                      }
                      frame "X-Y-Z stack" {
                        n3439 = call "2pparameters.vi"("command"="get") -> ("params out"=w102:T12)  [unwired: 1 in]
                        n3440 = Bundle By Name(cluster=w102, "type"="X-Y-Z stack") -> (w100:T12)
                        n3441 = call "2pparameters.vi"("Params in"=w100, "command"="set") -> ()  [unwired: 1 out]
                      }
                      frame "Lifetime (scan)" {
                        n3442 = call "2pparameters.vi"("command"="get") -> ("params out"=w107:T12)  [unwired: 1 in]
                        n3443 = Bundle By Name(cluster=w107, "type"="Lifetime (scan)") -> (w105:T12)
                        n3444 = call "2pparameters.vi"("Params in"=w105, "command"="set") -> ()  [unwired: 1 out]
                      }
                      frame "Lifetime (contour)" {
                        n3445 = local read "Vy-min draw"() -> (w117:dbl)
                        n3446 = local read "Vy-max draw"() -> (w116:dbl)
                        n3447 = local read "Vx-min draw"() -> (w119:dbl)
                        n3448 = local read "Vx-max draw"() -> (w118:dbl)
                        n3449 = local read "xpixels ref"() -> (w115:i32)
                        n3450 = local read "ypixels ref"() -> (w114:i32)
                        n3451 = local read "ROI Type"() -> (w113:u16)
                        n3452 = local read "srateAODOtt"() -> (w124:dbl)
                        n3453 = local read "# of frames"() -> (w129:i32)
                        n3454 = local read "refreshtime"() -> (w121:dbl)
                        n3455 = local read "Pel"() -> (w112:dbl)
                        n3456 = local read "bin"() -> (w127:dbl)
                        n3457 = local read "Override AI buffer"() -> (w110:bool)
                        n3458 = local read "finite samples"() -> (w136:bool)
                        n3459 = local read "srateAODOtt"() -> (w123:dbl)
                        n3460 = local read "srateAODOtt"() -> (w130:dbl)
                        n3461 = local read "continuous"() -> (w135:bool)
                        n3462 = local read "Angle ref"() -> (w120:dbl)
                        n3463 = local read "wavdet"() -> (w137:bool)
                        n3464 = local read "Vx-ref"() -> (w132:dbl)
                        n3465 = local read "Vy-ref"() -> (w134:dbl)
                        n3466 = local read "avpp"() -> (w133:i32)
                        n3467 = call "tt_timeandsamples.vi"("bin"=w127, "refreshtime"=w121, "srateAODOtt"=w124, "tot#ofsamples"=w129) -> ("refreshrate"=w125:dbl, "refreshbuffer"=w126:i32, "timetracecycles"=w131:i32)  [unwired: 5 in]
                        n3468 = local read "bin"() -> (w128:dbl)
                        n3469 = call "2pparameters.vi"("command"="get") -> ("params out"=w140:T12)  [unwired: 1 in]
                        n3470 = Bundle By Name(cluster=w140, "Drawing Mode"=w113, "measpoints"=w129, "tt_cycles"=w131, "refreshbuffer"=w126, "refreshrate"=w125, "Vx-ref"=w132, "Vy-ref"=w134, "srate"=w123, "finite"=w136, "cont"=w135, "wavdet"=w137, "avpp"=w133, "srateAODO"=w130, "bufferAI"=w126, "bin"=w128, "Angle Img"=w120, "Vxminref"=w119, "Vxmaxref"=w118, "Vyminref"=w117, "Vymaxref"=w116, "Xpixels Img"=w115, "Ypixels Img"=w114, "Pel"=w112, "Vz-reset"=0.0, "AIoverride"=w110, "type"="Lifetime (contour)") -> (w138:T12)
                        n3471 = Reciprocal(x=w125) -> (1/x=w122:dbl)
                        n3472 = local write "refreshtime"(w122) -> ()
                        n3473 = call "2pparameters.vi"("Params in"=w138, "command"="set") -> ()  [unwired: 1 out]
                      }
                      frame "X-Y-Z-t movie" {
                      }
                      frame "linescan" {
                      }
                      frame "Timetrace" {
                        n3474 = local read "Vy-min draw"() -> (w150:dbl)
                        n3475 = local read "Vy-max draw"() -> (w149:dbl)
                        n3476 = local read "Vx-min draw"() -> (w152:dbl)
                        n3477 = local read "Vx-max draw"() -> (w151:dbl)
                        n3478 = local read "xpixels ref"() -> (w148:i32)
                        n3479 = local read "ypixels ref"() -> (w147:i32)
                        n3480 = local read "ROI Type"() -> (w146:u16)
                        n3481 = local read "srateAODOtt"() -> (w157:dbl)
                        n3482 = local read "# of frames"() -> (w162:i32)
                        n3483 = local read "refreshtime"() -> (w154:dbl)
                        n3484 = local read "Pel"() -> (w145:dbl)
                        n3485 = local read "bin"() -> (w160:dbl)
                        n3486 = local read "Override AI buffer"() -> (w143:bool)
                        n3487 = local read "finite samples"() -> (w169:bool)
                        n3488 = local read "srateAODOtt"() -> (w156:dbl)
                        n3489 = local read "srateAODOtt"() -> (w163:dbl)
                        n3490 = local read "continuous"() -> (w168:bool)
                        n3491 = local read "Angle ref"() -> (w153:dbl)
                        n3492 = local read "wavdet"() -> (w170:bool)
                        n3493 = local read "Vx-ref"() -> (w165:dbl)
                        n3494 = local read "Vy-ref"() -> (w167:dbl)
                        n3495 = local read "avpp"() -> (w166:i32)
                        n3496 = call "tt_timeandsamples.vi"("bin"=w160, "refreshtime"=w154, "srateAODOtt"=w157, "tot#ofsamples"=w162) -> ("refreshrate"=w158:dbl, "refreshbuffer"=w159:i32, "timetracecycles"=w164:i32)  [unwired: 5 in]
                        n3497 = local read "bin"() -> (w161:dbl)
                        n3498 = call "2pparameters.vi"("command"="get") -> ("params out"=w173:T12)  [unwired: 1 in]
                        n3499 = Bundle By Name(cluster=w173, "Drawing Mode"=w146, "measpoints"=w162, "tt_cycles"=w164, "refreshbuffer"=w159, "refreshrate"=w158, "Vx-ref"=w165, "Vy-ref"=w167, "srate"=w156, "finite"=w169, "cont"=w168, "wavdet"=w170, "avpp"=w166, "srateAODO"=w163, "bufferAI"=w159, "bin"=w161, "Angle Img"=w153, "Vxminref"=w152, "Vxmaxref"=w151, "Vyminref"=w150, "Vymaxref"=w149, "Xpixels Img"=w148, "Ypixels Img"=w147, "Pel"=w145, "Vz-reset"=0.0, "AIoverride"=w143, "type"="Timetrace") -> (w171:T12)
                        n3500 = Reciprocal(x=w158) -> (1/x=w155:dbl)
                        n3501 = local write "refreshtime"(w155) -> ()
                        n3502 = call "2pparameters.vi"("Params in"=w171, "command"="set") -> ()  [unwired: 1 out]
                      }
                      frame "Lifetime (point)" {
                      }
                    }
                  }
                  frame #1 {
                    w176 = FALSE ("wavdet")
                    n3503 = call "2pparameters.vi"("command"="get") -> ("params out"=w180:T12)  [unwired: 1 in]
                    n3504 = Bundle By Name(cluster=w180, "finite"=w176, "cont"=w176, "wavdet"=TRUE) -> (w177:T12)
                    n3505 = call "2pparameters.vi"("Params in"=w177, "command"="set") -> ()  [unwired: 1 out]
                  }
                  frame #2 {
                    # "change active waveform numbers array"
                    n3506 = local read "AO channels"() -> (w187:u32)
                    n3507 = call "2pparameters.vi"("command"="get") -> ("params out"=w185:T12)  [unwired: 1 in]
                    n3508 = in-place {
                      in-place-border: w187 -> [w191]
                      in-place-border: [w188] -> w182
                      n3509 = in-place-cluster #49(w185) -> ("aAO"=w190:u32[])
                      n3510 = call "add channel to active arrayv2.vi"("line array in"=w190, "line to add"=w191) -> ("line array out"=w189:u32[], "addition"=w188:bool)  [unwired: 1 out]
                      n3511 = in-place-cluster #49("aAO"=w189) -> (w183:T12)
                    }
                    n3512 = local write "addAO"(w182) -> ()
                    n3513 = call "2pparameters.vi"("Params in"=w183, "command"="set") -> ()  [unwired: 1 out]
                  }
                  frame #3 {
                    # "update GUI"
                    n3514 = local read "addAO"() -> (w192:bool)
                    n3515 = case shown="True" w192 {
                      frame False {
                      }
                      frame True {
                        n3516 = call "Used AO lines.vi"() -> ("used AO names"=w196:string[], "used AO lines"=w198:tag[])  [unwired: 2 in]
                        n3517 = control-ref of="Analog Lines Plot"() -> (w197:refnum<vi>)
                        n3518 = control-ref of="Digital Lines Plot"() -> (w195:refnum<vi>)
                        n3519 = call "Used DO lines.vi"() -> ("used DO names"=w194:string[], "used DO lines"=w193:tag[])  [unwired: 2 in]
                        n3520 = local write "Analog Used Lines"(w198) -> ()
                        n3521 = local write "Analog Used Names"(w196) -> ()
                        n3522 = local write "Digital Used Lines"(w193) -> ()
                        n3523 = local write "Digital Used Names"(w194) -> ()
                        n3524 = call "prepDOWaveplot.vi"("DigitalGraph in"=w195, "used DO names"=w194) -> ()  [unwired: 1 in]
                        n3525 = call "prepAOWaveplot.vi"("WaveformGraph in"=w197, "Analog Used Names"=w196) -> ()  [unwired: 1 in]
                      }
                    }
                  }
                  frame #4 {
                    n3526 = local read "addAO"() -> (w199:bool)
                    n3527 = case shown="True" w199 {
                      frame False {
                      }
                      frame True {
                        # "add parameters\nto parameter array"
                        n3528 = local read "Build analog waveform tabs"() -> (w200:enum32{"Square", "Triangle", "Matlab"})
                        n3529 = case shown="\"Square\", Default" w200 {
                          frame "Square", Default {
                            w213 = 0.0 ("Offset (V)")
                            n3530 = local read "Meastab"() -> (w202:enum32{"X-Y Image", "Linescan", "Timetrace"})
                            n3531 = call "waveformparamsv2.vi"("command"="get") -> ("Params out"=w211:T16)  [unwired: 4 in, 2 out]
                            n3532 = Unbundle By Name(w211) -> ("AO parameters"=w208:T17)
                            n3533 = case shown="\"Timetrace\"" w202 {
                              tunnel: [w224 w225] -> w201
                              frame "X-Y Image", Default {
                                n3534 = local read "Sampling rate"() -> (w224:dbl)
                              }
                              frame "Timetrace" {
                                n3535 = local read "srateAODOtt"() -> (w225:dbl)
                              }
                            }
                            n3536 = local read "Start amplitude (V)"() -> (w221:dbl)
                            n3537 = local read "phase shift (ms)"() -> (w214:dbl)
                            n3538 = local read "Step size (V)"() -> (w219:dbl)
                            n3539 = local read "Baseline (V)"() -> (w220:dbl)
                            n3540 = local read "Period (ms)"() -> (w217:dbl)
                            n3541 = local read "padding value"() -> (w204:dbl)
                            n3542 = local read "Repeats"() -> (w223:dbl)
                            n3543 = local read "DC (%)"() -> (w218:dbl)
                            n3544 = local read "Cycles"() -> (w222:dbl)
                            n3545 = local read "Pulses"() -> (w215:dbl)
                            n3546 = Index Array(array=w208, index=0) -> (element=w209:T18)
                            n3547 = Bundle By Name(cluster=w209, "AOtab"=0.0 ("Repeats"), "Repeats"=w223, "Cycles"=w222, "Start amplitude (V)"=w221, "Baseline (V)"=w220, "Step size (V)"=w219, "DC (%)"=w218, "Sampling frequency (Hz)"=w201, "Period (ms)"=w217, "Offset (V)"=w213, "Amplitude (V)"=w213, "Frequency"=w213, "Tri Repeats"=w213, "phase shift (ms)"=w214, "Pulses"=w215, "Matlab wave file"=path "", "padding value"=w204) -> (w206:T18)
                            n3548 = Build Array(w206) -> (w205:T17)
                            n3549 = call "waveformparamsv2.vi"("command"="add AO", "add AO"=w205) -> ()  [unwired: 3 in, 3 out]
                          }
                          frame "Matlab" {
                            w231 = 0.0 ("Repeats")
                            n3550 = local read "Meastab"() -> (w227:enum32{"X-Y Image", "Linescan", "Timetrace"})
                            n3551 = call "waveformparamsv2.vi"("command"="get") -> ("Params out"=w238:T16)  [unwired: 4 in, 2 out]
                            n3552 = Unbundle By Name(w238) -> ("AO parameters"=w235:T17)
                            n3553 = case shown="\"Timetrace\"" w227 {
                              tunnel: [w241 w242] -> w226
                              frame "X-Y Image", Default {
                                n3554 = local read "Sampling rate"() -> (w241:dbl)
                              }
                              frame "Timetrace" {
                                n3555 = local read "srateAODOtt"() -> (w242:dbl)
                              }
                            }
                            n3556 = local read "Matlab waveform path"() -> (w228:path)
                            n3557 = local read "Matlab padding value"() -> (w230:dbl)
                            n3558 = Index Array(array=w235, index=0) -> (element=w236:T18)
                            n3559 = call "matlabwfexistsdialogue.vi"("Matlab waveform path"=w228) -> ("mtalab waveform path out"=w229:path)
                            n3560 = Bundle By Name(cluster=w236, "AOtab"=2.0 ("Repeats"), "Repeats"=w231, "Cycles"=w231, "Start amplitude (V)"=w231, "Baseline (V)"=w231, "Step size (V)"=w231, "DC (%)"=w231, "Sampling frequency (Hz)"=w226, "Period (ms)"=w231, "Offset (V)"=w231, "Amplitude (V)"=w231, "Frequency"=w231, "Tri Repeats"=w231, "phase shift (ms)"=w231, "Pulses"=w231, "Matlab wave file"=w229, "padding value"=w230) -> (w233:T18)
                            n3561 = Build Array(w233) -> (w232:T17)
                            n3562 = call "waveformparamsv2.vi"("command"="add AO", "add AO"=w232) -> ()  [unwired: 3 in, 3 out]
                          }
                          frame "Triangle" {
                            w248 = 0.0 ("Offset (V)")
                            n3563 = local read "Meastab"() -> (w244:enum32{"X-Y Image", "Linescan", "Timetrace"})
                            n3564 = call "waveformparamsv2.vi"("command"="get") -> ("Params out"=w260:T16)  [unwired: 4 in, 2 out]
                            n3565 = Unbundle By Name(w260) -> ("AO parameters"=w257:T17)
                            n3566 = case shown="\"Timetrace\"" w244 {
                              tunnel: [w262 w263] -> w243
                              frame "X-Y Image", Default {
                                n3567 = local read "Sampling rate"() -> (w262:dbl)
                              }
                              frame "Timetrace" {
                                n3568 = local read "srateAODOtt"() -> (w263:dbl)
                              }
                            }
                            n3569 = local read "Tri padding value"() -> (w246:dbl)
                            n3570 = local read "Amplitude (V)"() -> (w251:dbl)
                            n3571 = local read "Tri Phase (s)"() -> (w247:dbl)
                            n3572 = local read "Tri Repeats"() -> (w249:dbl)
                            n3573 = local read "Frequency"() -> (w250:dbl)
                            n3574 = local read "Offset (V)"() -> (w252:dbl)
                            n3575 = Index Array(array=w257, index=0) -> (element=w258:T18)
                            n3576 = Bundle By Name(cluster=w258, "AOtab"=1.0 ("Repeats"), "Repeats"=w248, "Cycles"=w248, "Start amplitude (V)"=w248, "Baseline (V)"=w248, "Step size (V)"=w248, "DC (%)"=w248, "Sampling frequency (Hz)"=w243, "Period (ms)"=w248, "Offset (V)"=w252, "Amplitude (V)"=w251, "Frequency"=w250, "Tri Repeats"=w249, "phase shift (ms)"=w248, "Pulses"=w248, "Matlab wave file"=path "", "Tri phase"=w247, "padding value"=w246) -> (w255:T18)
                            n3577 = Build Array(w255) -> (w254:T17)
                            n3578 = call "waveformparamsv2.vi"("command"="add AO", "add AO"=w254) -> ()  [unwired: 3 in, 3 out]
                          }
                        }
                      }
                    }
                  }
                  frame #5 {
                    n3579 = local read "addAO"() -> (w264:bool)
                    n3580 = case shown="True" w264 {
                      frame False {
                      }
                      frame True {
                        # "add waveform to waveform array; correct waveform lengths and plot"
                        n3581 = local read "Meastab"() -> (w268:enum32{"X-Y Image", "Linescan", "Timetrace"})
                        n3582 = local read "Build analog waveform tabs"() -> (w278:enum32{"Square", "Triangle", "Matlab"})
                        n3583 = case shown="\"Timetrace\"" w268 {
                          tunnel: [w286 w287] -> w267
                          frame "X-Y Image", Default {
                            n3584 = local read "Sampling rate"() -> (w286:dbl)
                          }
                          frame "Timetrace" {
                            n3585 = local read "srateAODOtt"() -> (w287:dbl)
                          }
                        }
                        n3586 = call "waveformparamsv2.vi"("command"="get last AO") -> ("last AO"=w280:T18)  [unwired: 4 in, 2 out]
                        n3587 = case shown="\"Matlab\"" w278 {
                          tunnel: w280 -> [w290 w292 w294]
                          tunnel: [w289 w291 w293] -> w279
                          frame "Square", Default {
                            n3588 = call "generateRampedSquareWave_fromAOparameters.vi"("AO params"=w290) -> ("Waveform"=w289:waveform(dbl))  [unwired: 1 out]
                          }
                          frame "Triangle" {
                            n3589 = call "generateTriWave_fromAOparameters.vi"("AO params"=w292) -> ("Waveform"=w291:waveform(dbl))  [unwired: 1 out]
                          }
                          frame "Matlab" {
                            n3590 = call "matlabAOwffromparam.vi"("Cluster"=w294) -> ("Waveform"=w293:waveform(dbl))  [unwired: 1 out]
                          }
                        }
                        n3591 = property on="refwf" class="Ring (strict)"() -> ("RingText.Text"=w271:string)  [unwired: 2 in, 2 out]
                        n3592 = call "waveformsAObuffer.vi"("command"="get") -> ("AO wf out"=w284:waveform(dbl)[])  [unwired: 1 in]
                        n3593 = Build Array (concatenate)(w284, w279) -> (w281:waveform(dbl)[])
                        n3594 = call "waveformsDObuffer.vi"("command"="get") -> ("DO wf out"=w276:digitalwaveform[])  [unwired: 1 in]
                        n3595 = call "correctwaveformsizetemp.vi"("new sampling frequency (Hz)"=w267, "start"=FALSE, "reference waveforms to"=w271, "Analog waveforms in"=w281, "stop"=FALSE, "Digital waveforms in"=w276) -> ("analog wf out"=w274:waveform(dbl)[], "Digital wf out"=w272:digitalwaveform[], "measpoints"=w269:i32)
                        n3596 = local write "Analog Lines Plot"(w274) -> ()
                        n3597 = call "GetNumCamFramesv2.vi"("Digital Waveform Graph"=w272) -> ("Numeric"=w273:i32)  [unwired: 10 in]
                        n3598 = local write "Digital Lines Plot"(w272) -> ()
                        n3599 = call "waveformsAObuffer.vi"("AO wf in"=w274, "command"="set") -> ()  [unwired: 1 out]
